vi "方程事件.vi"() -> ()   [LabVIEW 2018]
panel:
  in  "停止":bool
  in  "计算 2":bool
  in  "A 2":dbl
  in  "X 2":dbl
  in  "B 2":dbl
  in  "C 2":dbl
  out "结果 2":dbl
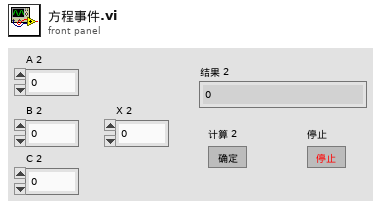
[diagram p1: front panel]
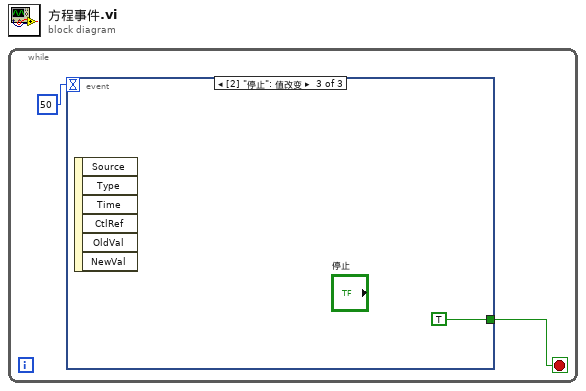
[diagram p0: block diagram]
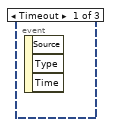
[diagram p2: hidden frame]
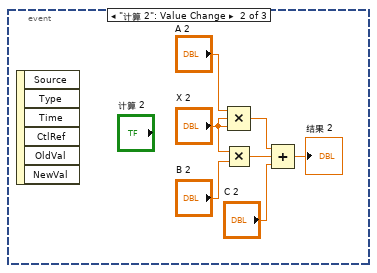
[diagram p3: hidden frame]
diagram:
  n1 = while {
    stop <- w1 stop-if-true
    n2 = event shown="[2] \"停止\": 值改变" {
      selector: _ -> [_ _ _]
      dyn-events: _ -> [_ _ _]
      timeout: 50 -> [_ _ _]
      tunnel: [_ _ TRUE] -> w1
      event Timeout {
        n3 = event-data() -> ()  [unwired: 1 in, 3 out]
      }
      event "计算 2": Value Change {
        n4 = event-data() -> ()  [unwired: 1 in, 6 out]
        n5 = Multiply(x="X 2", y="B 2") -> (x*y=w8:dbl)
        n6 = Compound Arithmetic op=MULTIPLY("A 2", "X 2", "X 2") -> (w7:dbl)
        n7 = Compound Arithmetic op=ADD(w7, w8, "C 2") -> (→"结果 2":dbl)
      }
      event "停止": Value Change {
        n8 = event-data() -> ()  [unwired: 1 in, 6 out]
      }
    }
  }
